vi "Configure.vi"(8 "error in (no error)":errorcluster, 11 "1553 Board in":refnum<class "1553 Session.lvclass">) -> (0 "error out":errorcluster, 3 "1553 Board out":refnum<class "1553 Session.lvclass">)   [LabVIEW 2020, in "BCI-1553 API.lvlib" / "1553 Session.lvclass"]
doc: "After a 1553 Session has been initialized, it must be configured. Configure will push the initialized parameters and settings to the BCI-1553 hardware and prepare it for running. This method must be called before the 'Start' method."
uses:
  1553 Session.lvclass
  1553 Session.lvclass/1553 Session.ctl
  1553 Component/1553 Component.lvclass
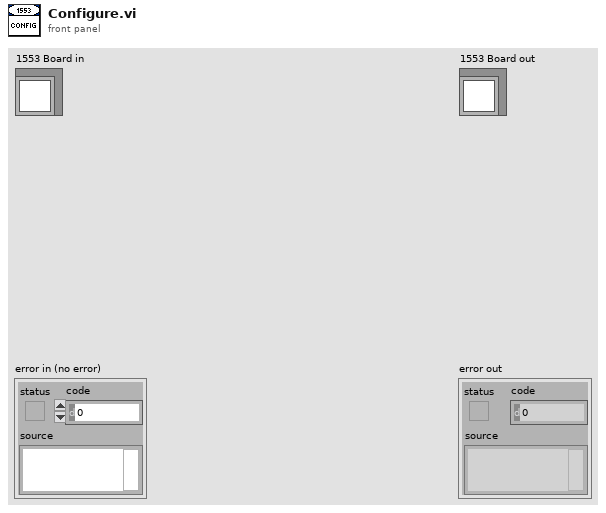
[diagram p1: front panel]
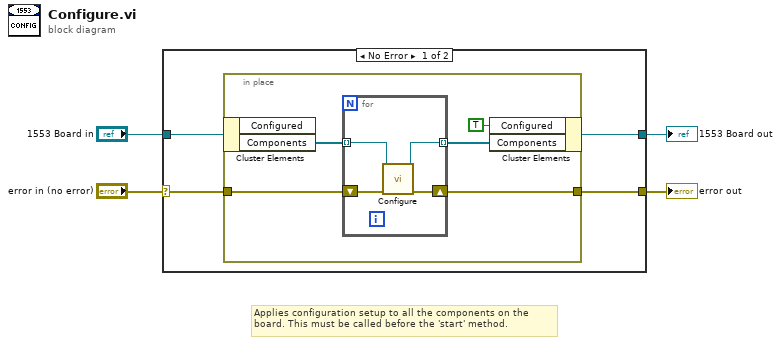
[diagram p0: block diagram]
diagram:
  # "Applies configuration setup to all the components on the\nboard. This must be called before the 'start' method."
  n1 = case shown="No Error" "error in (no error)" {
    selector: "error in (no error)" -> [w6 w19]
    tunnel: [w5 w19] -> w3
    tunnel: [w7 w18] -> w1
    tunnel: "1553 Board in" -> [w8 w18]
    frame No Error {
      n2 = in-place {
        in-place-border: w6 -> [w11]
        in-place-border: [w10] -> w5
        n3 = in-place-cluster #1(w8) -> ("Components"=w13:refnum<class "1553 Component.lvclass">[])  [unwired: 1 out]
        n4 = for {
          tunnel: w13 -> [w17] mode=indexing
          tunnel: [w16] -> w12 mode=indexing
          shift-right: [w14] -> w10
          shift-left: w11 -> [w15]
          n5 = call-dynamic "Configure.vi"("error in (no error)"=w15, "1553 Component in"=w17) -> ("error out"=w14:errorcluster, "1553 Component out"=w16:refnum<class "1553 Component.lvclass">)  [unwired: 8 in]
        }
        n6 = in-place-cluster #1("Configured"=TRUE, "Components"=w12) -> (w7:refnum<class "1553 Session.lvclass">)
      }
    }
    frame Error {
    }
  }
  "error out" <- w3
  "1553 Board out" <- w1
